vi "MicroPulse - determine data retention.vi"(5 "retain scan":T1) -> (2 "retain scan":T1)   [LabVIEW 2026, in "MicroPulse_Driver.lvlib"]
uses:
  MicroPulse_Driver.lvlib
  Public/Data/Datatypes/MP - retain scan.ctl
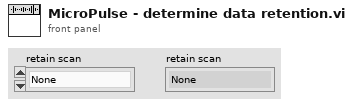
[diagram p1: front panel]
types:
  T1 = typedef "MicroPulse_Driver.lvlib/MP - retain scan.ctl" = enum16{"None", "Ascan", "Peaks"}
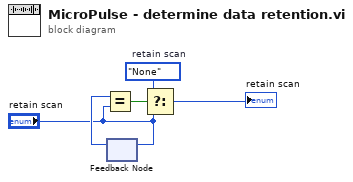
[diagram p0: block diagram]
diagram:
  w2 = MP_-_retain_scan."None"  # retain scan
  n1 = feedback #1() -> (w4:T1)  [unwired: 1 in]
  n2 = Equal?(x=w4, y="retain scan") -> (x = y?=w5:bool)
  n3 = feedback-in #1("retain scan") -> ()
  n4 = Select(t=w2, s=w5, f="retain scan") -> (s? t:f=→"retain scan":T1)
